vi "DistanceSensorGetSonarReflections.vi"(0 "Device In":u64, 11 "error in (no error)":errorcluster) -> (4 "Device Out":u64, 6 "Distances":u32[](array[numeric]), 8 "Amplitudes":u32[](array[numeric]), 10 "Count":u32, 15 "error out":errorcluster)   [LabVIEW 2012, in "Phidget Distance Sensor.lvlib"]
doc: "${GetSonarReflections:Header}"
uses:
  <instrlib>/Phidgets/Phidget Distance Sensor/Phidget Distance Sensor.lvlib
  <instrlib>/Phidgets/Phidget Common/Phidget Common.lvlib
  phidget22.dll
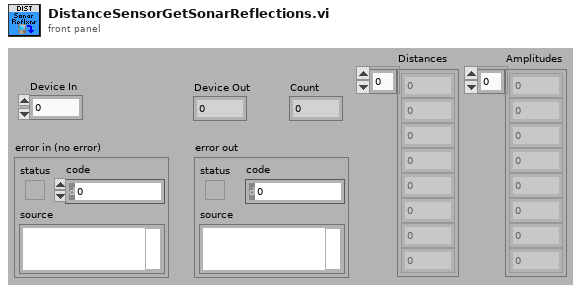
[diagram p1: front panel]
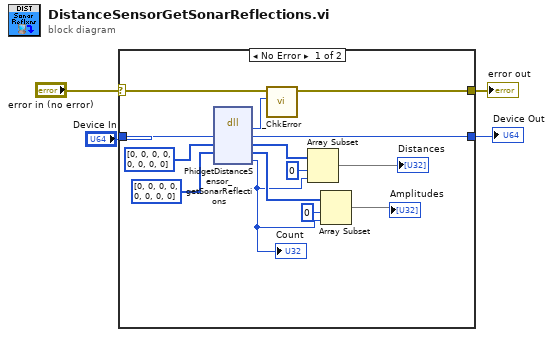
[diagram p0: block diagram]
diagram:
  n1 = case shown="No Error" "error in (no error)" {
    selector: "error in (no error)" -> [w16 w20]
    tunnel: [w15 w20] -> w3
    tunnel: "Device In" -> [w18 w19]
    tunnel: [w17 w19] -> w2
    frame No Error {
      n2 = dll-call lib="phidget22.*" fn="PhidgetDistanceSensor_getSonarReflections"("phid"=w18, "distances"=u32[] [0, 0, 0, 0, 0, 0, 0, 0], "amplitudes"=u32[] [0, 0, 0, 0, 0, 0, 0, 0]) -> ("return type"=w14:i32, "phid"=w17:u64, "distances"=w10:u32[], "amplitudes"=w7:u32[], "count"=w5:u32)  [unwired: 4 in, 2 out]
      "Count" <- w5
      n3 = call <instrlib>:"_ChkError.vi"("Return Code"=w14, "error in (no error)"=w16) -> ("error out"=w15:errorcluster)  [unwired: 9 in]
      n4 = Array Subset(array=w10, index=0, length=w5) -> (→"Distances":u32[])
      n5 = Array Subset(array=w7, index=0, length=w5) -> (→"Amplitudes":u32[])
    }
    frame Error {
    }
  }
  "error out" <- w3
  "Device Out" <- w2
